vi "Test Set Row Values DBL.vi"(11 "Test Case In":refnum<class "Test Open Xml.lvclass">) -> (0 "error out":errorcluster, 3 "Test Case Out":refnum<class "Test Open Xml.lvclass">)   [LabVIEW 2020, in "Test Open Xml.lvclass"]
uses:
  Test Open Xml.lvclass
  <vilib>/Astemes/LUnit/Test Case.lvclass
  Source/Open Xml.lvlib
  Source/Cell DataType.ctl
  e5169541-515f-4f16-96fe-0f2d3de234a9.vi
  c685489d-b27d-4ca7-9de3-cc8e1658789f.vi
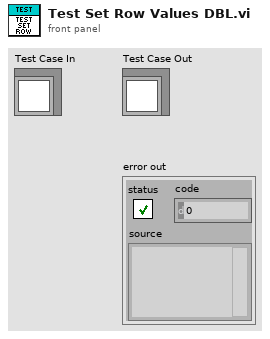
[diagram p1: front panel]
types:
  T1 = typedef "Open Xml.lvlib/Cell DataType.ctl" = enum16{"Void", "Boolean", "Number", "Error", "SharedString", "String", "InlineString", "Date"}
  T2 = cluster{"Number":dbl, "String":string, "Boolean":bool, "Time Stamp":timestamp, "Error":errorcluster}[]
  T3 = cluster{"Number":dbl, "String":string, "Boolean":bool, "Time Stamp":timestamp, "Error":errorcluster}
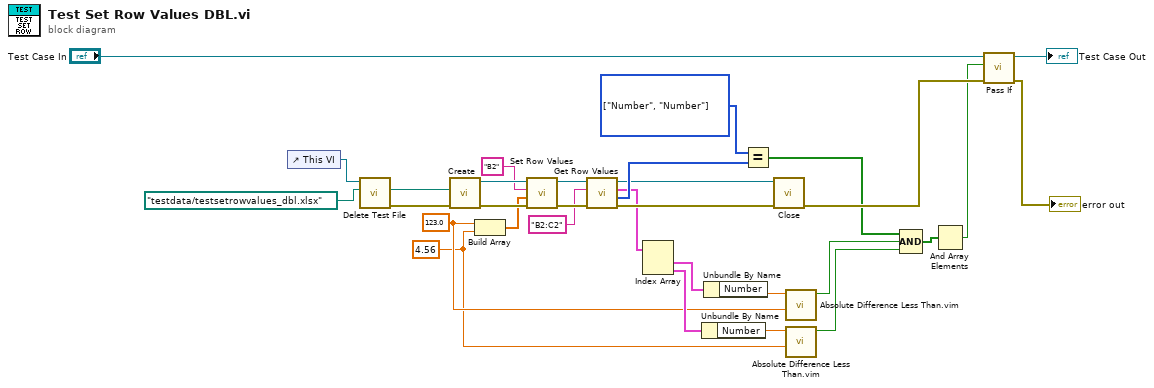
[diagram p0: block diagram]
diagram:
  w16 = T1[] [enum."Number", enum."Number"] items=["Void", "Boolean", "Number", "Error", "SharedString", "String", "InlineString", "Date"] ("x")
  w6 = 4.56
  w7 = 123.0
  n1 = control-ref of="This VI"() -> (w2:refnum<vi>)
  n2 = call "Delete Test File.vi"("name or relative path"=path "testdata/testsetrowvalues_dbl.xlsx", "VI in"=w2) -> ("error out"=w4:errorcluster, "deleted path"=w3:path)  [unwired: 8 in]
  n3 = call "Create.vi"("error in"=w4, "Path"=w3) -> ("error out"=w27:errorcluster, "SpreadsheetDoc"=w28:refnum<k24>)  [unwired: 8 in]
  n4 = Build Array(w7, w6) -> (w11:dbl[])
  n5 = call "Set Row Values.vi"("error in"=w27, "Values"=w11, "Cell Address"="B2", "SpreadsheetDoc"=w28) -> ("error out"=w23:errorcluster, "SpreadsheetDoc out"=w22:refnum<k24>)  [unwired: 6 in]
  n6 = call "Get Row Values.vi"("error in"=w23, "Cell Addresses"="B2:C2" ("Cell Address"), "SpreadsheetDoc in"=w22) -> ("error out"=w25:errorcluster, "Types"=w21:T1[], "Cell Values"=w17:T2, "SpreadsheetDoc out"=w5:refnum<k24>)  [unwired: 5 in]
  n7 = Index Array(array=w17) -> (element #1=w15:T3, element #2=w14:T3)  [unwired: 2 in]
  n8 = Unbundle By Name(w14) -> ("Number"=w9:dbl)
  n9 = Unbundle By Name(w15) -> ("Number"=w12:dbl)
  n10 = Equal?(x=w16, y=w21) -> (x = y?=w20:bool[])
  n11 = call "Close.vi"("error in"=w25, "SpreadsheetDoc"=w5) -> ("error out"=w26:errorcluster)  [unwired: 9 in]
  n12 = call "Absolute Difference Less Than.vim"("Number 2"=w7, "Number 1"=w12) -> ("In Limit"=w8:bool)  [unwired: 9 in]
  n13 = call "Absolute Difference Less Than.vim"("Number 2"=w6, "Number 1"=w9) -> ("In Limit"=w10:bool)  [unwired: 9 in]
  n14 = Compound Arithmetic op=AND(w20, w8, w10) -> (w13:bool[])
  n15 = And Array Elements(Boolean array=w13) -> (logical AND=w24:bool)
  n16 = call <vilib>:"Pass If.vi"("error in (no error)"=w26, "Pass?"=w24, "LUnit Test Case In"="Test Case In") -> ("error out"=→"error out":errorcluster, "LUnit Test Case Out"=→"Test Case Out":refnum<class "Test Open Xml.lvclass">)  [unwired: 7 in]
